vi "find_circles.vi"(5 "shrinkFactor":i32, 6 "Field of View":cluster{"fieldOfViewX":sgl, "fieldOfViewY":sgl}, 7 "logFileDir":string, 8 "error in":errorcluster, 9 "debug":bool, 10 "find_circles parameters":T2, 11 "Image":T3) -> (0 "error out":errorcluster, 2 "Circles":T1(array[cluster]))   [LabVIEW 2017, in "gVision.lvlib"]
uses:
  gVision.lvlib
  Vision.lvlib
  <vilib>/vision/Image Controls.llb/IMAQ Image.ctl
  find_circles parameters.ctl
panel:
  # "Image must be an 8-bin greyscale image"
  # "For error circle"
  # "in micrometers"
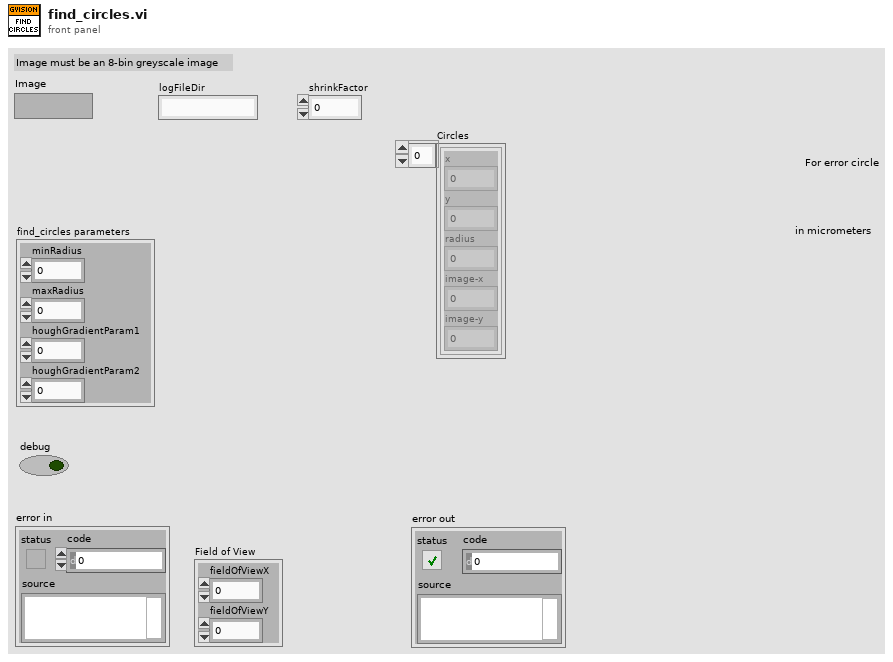
[diagram p1: front panel]
types:
  T1 = cluster{"x":dbl, "y":dbl, "radius":dbl, "image-x":dbl, "image-y":dbl}[]
  T2 = typedef "Vision.lvlib/find_circles parameters.ctl" = cluster{"minRadius":sgl, "maxRadius":sgl, "houghGradientParam1":i32, "houghGradientParam2":i32}
  T3 = typedef "IMAQ Image.ctl" = refnum<image>
  T4 = enum32{"Map Pixel Pointer", "Unmap Pixel Pointer", "Get Pixels Infos"}
  T5 = cluster{"x":dbl, "y":dbl, "radius":dbl, "image-x":dbl, "image-y":dbl}
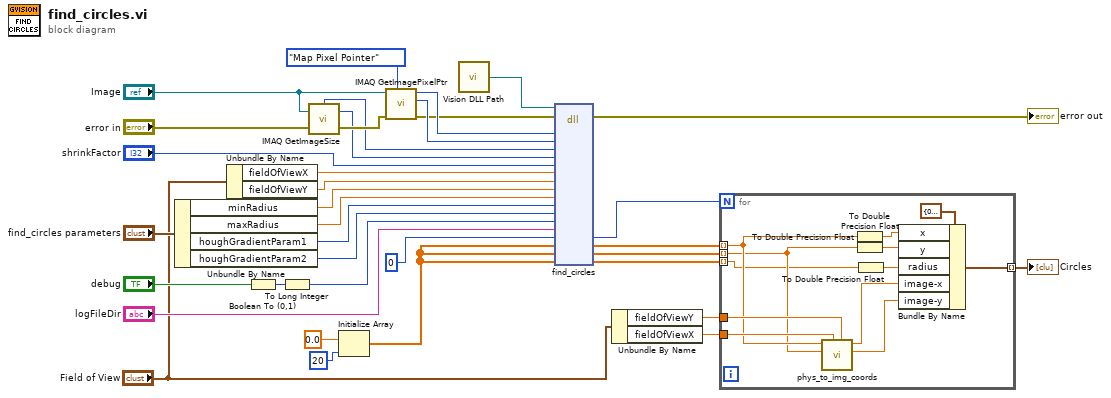
[diagram p0: block diagram]
diagram:
  n1 = Unbundle By Name("find_circles parameters") -> ("minRadius"=w23:sgl, "maxRadius"=w22:sgl, "houghGradientParam1"=w21:i32, "houghGradientParam2"=w20:i32)
  n2 = Unbundle By Name("Field of View") -> ("fieldOfViewX"=w3:sgl, "fieldOfViewY"=w2:sgl)
  n3 = Boolean To (0,1)(Boolean="debug") -> (0, 1=w24:i16)
  n4 = To Long Integer(number=w24) -> (32bit integer=w19:i32)
  n5 = call "IMAQ GetImageSize"("Image"="Image", "error in (no error)"="error in") -> ("Y Resolution"=w30:i32, "X Resolution"=w29:i32, "error out"=w31:errorcluster)  [unwired: 2 in]
  n6 = Initialize Array(sgl 0.0 ("element"), 20 ("dimension size")) -> (w15:sgl[])
  n7 = call "IMAQ GetImagePixelPtr"("Function"=T4."Map Pixel Pointer", "error in (no error)"=w31, "Image"="Image") -> ("error out"=w1:errorcluster, "LineWidth(Pixels)"=w28:i32, "Pixel Pointer out"=w27:u64)  [unwired: 3 in, 3 out]
  n8 = call "Vision DLL Path.vi"() -> ("DLL Path"=w35:path)  [unwired: 5 in]
  n9 = dll-call lib="?" fn="find_circles"(path in=w35, error in=w1, "img"=w27, "imgLineWidth"=w28, "imgWidth"=w29, "imgHeight"=w30, "shrinkFactor"="shrinkFactor", "fieldOfViewX"=w3, "fieldOfViewY"=w2, "minRadius"=w23, "maxRadius"=w22, "houghGradientParam1"=w21, "houghGradientParam2"=w20, "debug"=w19, "logFileDir"="logFileDir", "numCircles"=0, "circleXCenters"=w15, "circleYCenters"=w15, "circleRadii"=w15) -> (error out=→"error out":errorcluster, "numCircles"=w10:i32, "circleXCenters"=w9:sgl[], "circleYCenters"=w8:sgl[], "circleRadii"=w7:sgl[])  [unwired: 15 in, 1 out]
  n10 = Unbundle By Name("Field of View") -> ("fieldOfViewY"=w13:sgl, "fieldOfViewX"=w12:sgl)
  n11 = for {
    N: w10 -> [_]
    tunnel: w9 -> [w40] mode=indexing
    tunnel: w8 -> [w37] mode=indexing
    tunnel: [w47] -> w6 mode=indexing
    tunnel: w13 -> [w42]
    tunnel: w12 -> [w41]
    tunnel: w7 -> [w36] mode=indexing
    n12 = call "phys_to_img_coords.vi"("fov_y"=w42, "fov_x"=w41, "y"=w37, "x"=w40) -> ("image_y"=w38:dbl, "image_x"=w39:dbl)  [unwired: 6 in]
    n13 = To Double Precision Float(number=w40) -> (double precision float=w46:dbl)
    n14 = To Double Precision Float(number=w37) -> (double precision float=w45:dbl)
    n15 = To Double Precision Float(number=w36) -> (double precision float=w44:dbl)
    n16 = Bundle By Name(cluster=T5 {"x"=0.0, "y"=0.0, "radius"=0.0, "image-x"=0.0, "image-y"=0.0}, "x"=w46, "y"=w45, "radius"=w44, "image-x"=w39, "image-y"=w38) -> (w47:T5)
  }
  "Circles" <- w6
